vi "3.11-Select Critical Point.vi"(2 "Y (mm)":dbl[](array[numeric])=[-824.0, -821.8748054185536, -817.5016965016204, -818.8762184987505, -802.0414964088986, -800.9405372657634, -800.59012577146, -788.0816444032098, -786.2728465808068, -784.2245424325394, -781.9373558916932, -787.2650011250265, -784.474375788512, -778.521681763403, -776.2365810207972, -783.3658451204344, 730.5588889131224, 725.4102955430903, 724.8109075281693, 724.931328200215, 718.9384865393471, 714.6245895498994, 721.8640829579484, 720.0248002938554, 725.866494387571, 726.5437830014478, 731.9681149910491, 736.1878818898, 736.2022690917503, 745.9762624616667, 740.54860282115, 736.8877513302604, 737.0, -580.0, -600.0, -620.0, -640.0, -660.0, -680.0, -700.0, -720.0, -740.0, -760.0, -780.0, -800.0, -820.0, -840.0, -860.0, -880.0, -900.0, -920.0, -940.0, -960.0, -980.0, -1000.0, -1020.0, -1040.0, -1060.0, -1080.0, -1100.0, -1120.0, -1140.0, -1160.0, 580.0, 600.0, 620.0, 640.0, 660.0, 680.0, 700.0, 720.0, 740.0, 760.0, 780.0, 800.0, 820.0, 840.0, 860.0, 880.0, 900.0, 920.0, 940.0, 960.0, 980.0, 1000.0, 1020.0, 1040.0, 1060.0, 1080.0, 1100.0, 1120.0, 1140.0, 1160.0], 3 "X (mm)":dbl[](array[numeric])=[840.0, 854.3458780914469, 868.5477883026458, 882.9154841192139, 896.0842048902769, 910.0732171691171, 924.145412930461, 936.7642586636871, 950.5034421622921, 964.2089652419434, 977.8766530675427, 993.028814291989, 1006.7451760358431, 1019.7358924207481, 1033.5375164797342, 1049.9022455781442, 1049.4843904209192, 1034.373102871993, 1020.7156560129519, 1007.3635844318354, 992.8150927510532, 978.9089486341247, 967.2841142298599, 954.0407250143282, 942.0138830037281, 929.2083593725679, 916.9329489649929, 904.4080938905194, 891.4802776231645, 879.0949593134791, 865.8605270565532, 852.8624235442778, 840.0, 0.0, 0.0, 0.0, 0.0, 0.0, 0.0, 0.0, 0.0, 0.0, 0.0, 0.0, 0.0, 0.0, 0.0, 0.0, 0.0, 0.0, 0.0, 0.0, 0.0, 0.0, 0.0, 0.0, 0.0, 0.0, 0.0, 0.0, 0.0, 0.0, 0.0, 0.0, 0.0, 0.0, 0.0, 0.0, 0.0, 0.0, 0.0, 0.0, 0.0, 0.0, 0.0, 0.0, 0.0, 0.0, 0.0, 0.0, 0.0, 0.0, 0.0, 0.0, 0.0, 0.0, 0.0, 0.0, 0.0, 0.0, 0.0, 0.0, 0.0]) -> (0 "Left Data":T2, 1 "Right Data":T1)   [LabVIEW 2010]
panel:
  in  "Y (mm) 2":dbl[](array[numeric])
  in  "X (mm) 2":dbl[](array[numeric])
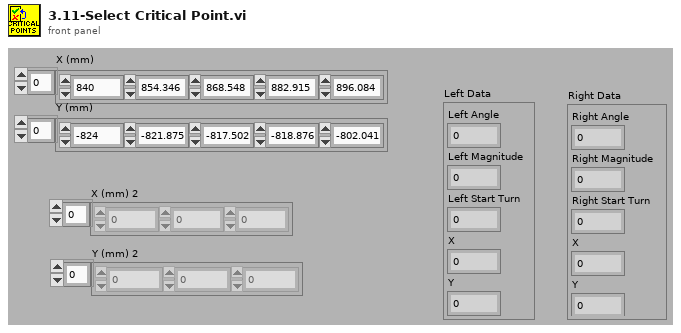
[diagram p1: front panel]
types:
  T1 = cluster{"Right Angle":dbl, "Right Magnitude":dbl, "Right Start Turn":dbl, "X":dbl, "Y":dbl}
  T2 = cluster{"Left Angle":dbl, "Left Magnitude":dbl, "Left Start Turn":dbl, "X":dbl, "Y":dbl}
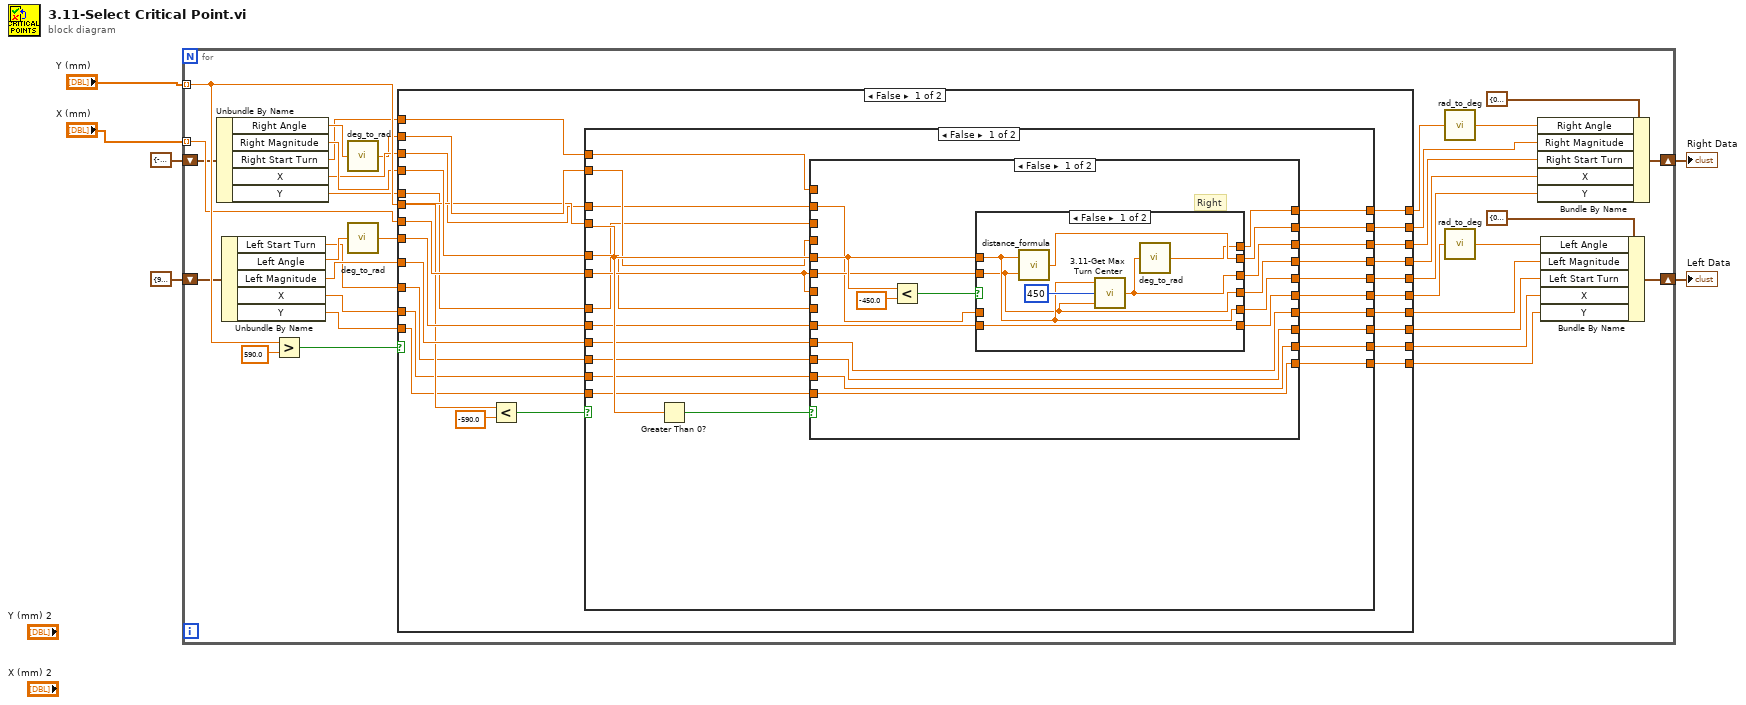
[diagram p0: block diagram]
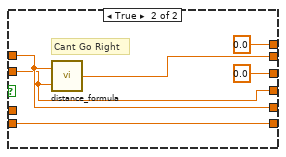
[diagram p2: hidden frame]
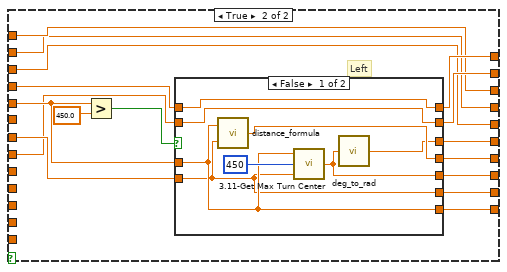
[diagram p3: hidden frame]
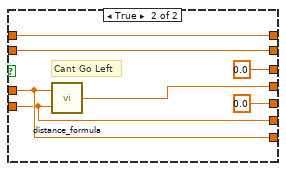
[diagram p4: hidden frame]
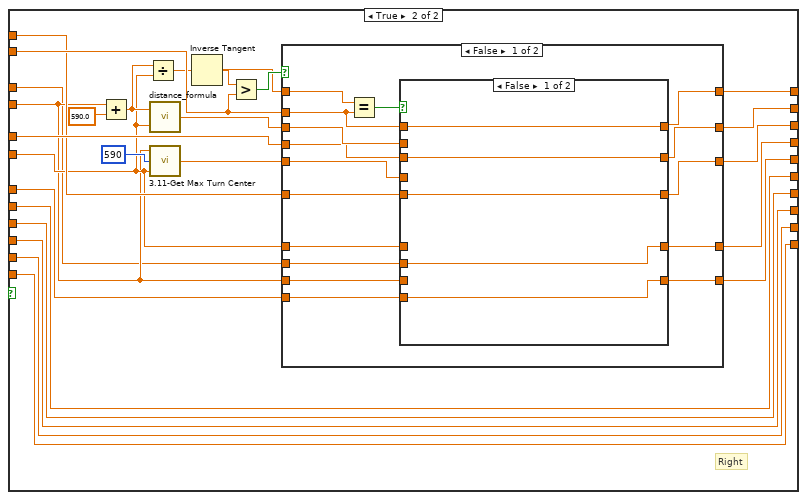
[diagram p5: hidden frame]
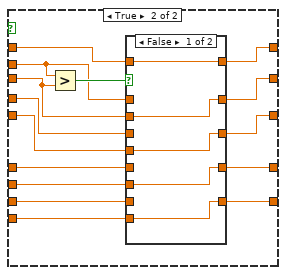
[diagram p6: hidden frame]
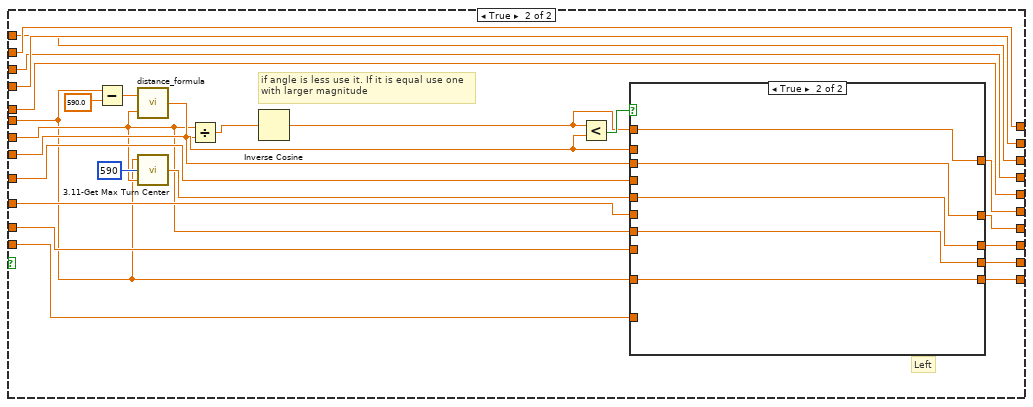
[diagram p9: hidden frame]
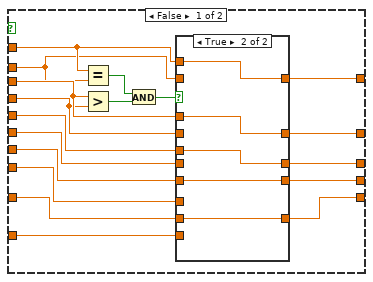
[diagram p10: hidden frame]
diagram:
  n1 = for {
    tunnel: "Y (mm)" -> [w38] mode=indexing
    tunnel: "X (mm)" -> [w37] mode=indexing
    shift-right: [w35] -> w3
    shift-left: T1 {"Right Angle"=-90.0, "Right Magnitude"=0.0, "Right Start Turn"=-90.0, "X"=-1.0, "Y"=-1701.0} ("input cluster") -> [w23]
    shift-right: [w21] -> w4
    shift-left: T2 {"Left Angle"=90.0, "Left Magnitude"=0.0, "Left Start Turn"=90.0, "X"=-1.0, "Y"=1701.0} ("input cluster") -> [w25]
    n2 = Unbundle By Name(w23) -> ("Right Angle"=w12:dbl, "Right Magnitude"=w22:dbl, "Right Start Turn"=w7:dbl, "X"=w15:dbl, "Y"=w13:dbl)
    n3 = Unbundle By Name(w25) -> ("Left Start Turn"=w8:dbl, "Left Angle"=w10:dbl, "Left Magnitude"=w24:dbl, "X"=w20:dbl, "Y"=w17:dbl)
    n4 = Greater?(x=w38, y=590.0) -> (0:w40:bool)
    n5 = call "deg_to_rad.vi"("Degrees"=w12) -> ("Radians"=w11:dbl)
    n6 = call "deg_to_rad.vi"("Degrees"=w10) -> ("Radians"=w9:dbl)
    n7 = case shown="False" w40 {
      tunnel: w38 -> [w53 w227]
      tunnel: w37 -> [w54 w229]
      tunnel: w9 -> [w62 w245]
      tunnel: [w61 w247] -> w29
      tunnel: [w59 w246] -> w26
      tunnel: w24 -> [w60 w244]
      tunnel: w11 -> [w58 w243]
      tunnel: [w57 w243] -> w32
      tunnel: [w55 w242] -> w33
      tunnel: w22 -> [w56 w242]
      tunnel: w8 -> [w49 w233]
      tunnel: [w50 w234] -> w27
      tunnel: [w52 w236] -> w34
      tunnel: w7 -> [w51 w236]
      tunnel: w20 -> [w42 w231]
      tunnel: [w41 w230] -> w19
      tunnel: [w44 w228] -> w18
      tunnel: w17 -> [w43 w226]
      tunnel: [w48 w225] -> w16
      tunnel: w15 -> [w47 w225]
      tunnel: [w46 w224] -> w14
      tunnel: w13 -> [w45 w224]
      frame False {
        n8 = Less?(x=w53, y=-590.0) -> (x < y?=w64:bool)
        n9 = case shown="False" w64 {
          tunnel: w62 -> [w83 w171]
          tunnel: [w85 w171] -> w61
          tunnel: w60 -> [w75 w170]
          tunnel: [w84 w170] -> w59
          tunnel: w58 -> [w79 w169]
          tunnel: [w82 w168] -> w57
          tunnel: w56 -> [w78 w166]
          tunnel: [w80 w167] -> w55
          tunnel: w54 -> [w81 w153]
          tunnel: w53 -> [w86 w152]
          tunnel: [w76 w159] -> w52
          tunnel: w51 -> [w73 w158]
          tunnel: [w77 w157] -> w50
          tunnel: w49 -> [w74 w157]
          tunnel: [w66 w155] -> w48
          tunnel: w47 -> [w72 w150]
          tunnel: [w67 w154] -> w46
          tunnel: w45 -> [w65 w151]
          tunnel: [w68 w148] -> w44
          tunnel: w43 -> [w69 w148]
          tunnel: [w71 w149] -> w41
          tunnel: w42 -> [w70 w149]
          frame False {
            n10 = Greater Than 0?(x=w86) -> (x > 0?=w87:bool)
            n11 = case shown="False" w87 {
              tunnel: w86 -> [w98 w129]
              tunnel: [w101 w130] -> w85
              tunnel: w81 -> [_ w128]
              tunnel: [w94 w127] -> w84
              tunnel: w83 -> [w100 _]
              tunnel: [w99 w126] -> w82
              tunnel: w81 -> [w97 _]
              tunnel: [w96 w124] -> w80
              tunnel: w79 -> [_ w125]
              tunnel: w78 -> [_ w123]
              tunnel: [w93 w122] -> w77
              tunnel: [w95 w121] -> w76
              tunnel: w75 -> [w94 _]
              tunnel: w74 -> [w93 _]
              tunnel: w73 -> [_ w121]
              tunnel: [w88 w117] -> w66
              tunnel: [w89 w118] -> w67
              tunnel: w72 -> [w92 w117]
              tunnel: [w91 w119] -> w71
              tunnel: w70 -> [w91 _]
              tunnel: w69 -> [w90 _]
              tunnel: [w90 w120] -> w68
              tunnel: w65 -> [_ w118]
              frame False {
                # "Right"
                n12 = Less?(x=w98, y=-450.0) -> (x < y?=w102:bool)
                n13 = case shown="False" w102 {
                  tunnel: [w109 w116] -> w101
                  tunnel: w100 -> [w109 w116]
                  tunnel: [w106 0.0 ("y")] -> w99
                  tunnel: w98 -> [w105 w112]
                  tunnel: w97 -> [w104 w111]
                  tunnel: [w108 w114] -> w96
                  tunnel: [w107 0.0 ("y")] -> w95
                  tunnel: w92 -> [_ _]
                  tunnel: [w105 w112] -> w89
                  tunnel: [w104 w111] -> w88
                  frame False {
                    n14 = call "distance_formula.vi"("X2 - X1"=w104, "Y2 - Y1"=w105) -> ("Distance"=w108:dbl)
                    n15 = call "3.11-Get Max Turn Center.vi"("X (mm)"=w104, "Distance Along Y where polar system is centered"=450, "Y (mm)"=w105) -> ("Start Turn Angle"=w107:dbl)
                    n16 = call "deg_to_rad.vi"("Degrees"=w107) -> ("Radians"=w106:dbl)
                  }
                  frame True {
                    # "Cant Go Right"
                    n17 = call "distance_formula.vi"("X2 - X1"=w111, "Y2 - Y1"=w112) -> ("Distance"=w114:dbl)
                  }
                }
              }
              frame True {
                # "Left"
                n18 = Greater?(x=w129, y=450.0) -> (0:w132:bool)
                n19 = case shown="False" w132 {
                  tunnel: [w135 0.0 ("y")] -> w130
                  tunnel: w129 -> [w134 w142]
                  tunnel: w128 -> [w133 w141]
                  tunnel: [w137 w146] -> w127
                  tunnel: [w139 w145] -> w126
                  tunnel: w125 -> [w139 w145]
                  tunnel: [w138 w144] -> w124
                  tunnel: w123 -> [w138 w144]
                  tunnel: [w136 0.0 ("y")] -> w122
                  tunnel: [w134 w142] -> w120
                  tunnel: [w133 w141] -> w119
                  frame False {
                    n20 = call "distance_formula.vi"("X2 - X1"=w133, "Y2 - Y1"=w134) -> ("Distance"=w137:dbl)
                    n21 = call "3.11-Get Max Turn Center.vi"("X (mm)"=w133, "Distance Along Y where polar system is centered"=450, "Y (mm)"=w134) -> ("Start Turn Angle"=w136:dbl)
                    n22 = call "deg_to_rad.vi"("Degrees"=w136) -> ("Radians"=w135:dbl)
                  }
                  frame True {
                    # "Cant Go Left"
                    n23 = call "distance_formula.vi"("X2 - X1"=w141, "Y2 - Y1"=w142) -> ("Distance"=w146:dbl)
                  }
                }
              }
            }
          }
          frame True {
            # "Right"
            n24 = Add(x=w152, y=590.0) -> (x+y=w162:dbl)
            n25 = Divide(x=w162, y=w153) -> (x/y=w163:dbl)
            n26 = call "distance_formula.vi"("X2 - X1"=w153, "Y2 - Y1"=w162) -> ("Distance"=w164:dbl)
            n27 = call "3.11-Get Max Turn Center.vi"("X (mm)"=w153, "Distance Along Y where polar system is centered"=590, "Y (mm)"=w152) -> ("Start Turn Angle"=w160:dbl)
            n28 = Inverse Tangent(1:w163) -> (0:w161:dbl)
            n29 = Greater?(x=w161, y=w169) -> (0:w172:bool)
            n30 = case shown="False" w172 {
              tunnel: w169 -> [w186 _]
              tunnel: w164 -> [w187 w223]
              tunnel: [w185 w222] -> w168
              tunnel: [w184 w223] -> w167
              tunnel: w166 -> [w183 _]
              tunnel: w161 -> [w182 w222]
              tunnel: [w181 w221] -> w159
              tunnel: w160 -> [w179 w221]
              tunnel: w158 -> [w180 _]
              tunnel: [w178 w220] -> w155
              tunnel: w153 -> [w177 w220]
              tunnel: [w176 w219] -> w154
              tunnel: w152 -> [w175 w219]
              tunnel: w151 -> [w174 _]
              tunnel: w150 -> [w173 _]
              frame False {
                n31 = Equal?(x=w182, y=w186) -> (x = y?=w188:bool)
                n32 = case shown="False" w188 {
                  tunnel: w187 -> [_ w203]
                  tunnel: w183 -> [w193 w207]
                  tunnel: w186 -> [w192 w206]
                  tunnel: [w192 w205] -> w185
                  tunnel: [w193 w204] -> w184
                  tunnel: [w191 w201] -> w181
                  tunnel: w180 -> [w191 w200]
                  tunnel: w179 -> [_ w202]
                  tunnel: [w189 w199] -> w178
                  tunnel: w177 -> [_ w198]
                  tunnel: [w190 w197] -> w176
                  tunnel: w175 -> [_ w196]
                  tunnel: w174 -> [w190 w195]
                  tunnel: w173 -> [w189 w194]
                  frame False {
                  }
                  frame True {
                    n33 = Greater?(x=w203, y=w207) -> (0:w208:bool)
                    n34 = case shown="False" w208 {
                      tunnel: w207 -> [w212 _]
                      tunnel: w206 -> [w213 w217]
                      tunnel: [w213 w217] -> w205
                      tunnel: [w212 w218] -> w204
                      tunnel: w203 -> [_ w218]
                      tunnel: [w211 w216] -> w201
                      tunnel: w202 -> [_ w216]
                      tunnel: w200 -> [w211 _]
                      tunnel: [w209 w215] -> w199
                      tunnel: w198 -> [_ w215]
                      tunnel: [w210 w214] -> w197
                      tunnel: w196 -> [_ w214]
                      tunnel: w195 -> [w210 _]
                      tunnel: w194 -> [w209 _]
                      frame False {
                      }
                      frame True {
                      }
                    }
                  }
                }
              }
              frame True {
              }
            }
          }
        }
      }
      frame True {
        # "if angle is less use it. If it is equal use one\nwith larger magnitude"
        # "Left"
        n35 = Subtract(x=w227, y=590.0) -> (x-y=w240:dbl)
        n36 = call "distance_formula.vi"("X2 - X1"=w229, "Y2 - Y1"=w240) -> ("Distance"=w238:dbl)
        n37 = call "3.11-Get Max Turn Center.vi"("X (mm)"=w229, "Distance Along Y where polar system is centered"=590, "Y (mm)"=w227) -> ("Start Turn Angle"=w235:dbl)
        n38 = Divide(x=w229, y=w238) -> (x/y=w239:dbl)
        n39 = Inverse Cosine(1:w239) -> (0:w237:dbl)
        n40 = Less?(x=w237, y=w245) -> (x < y?=w248:bool)
        n41 = case shown="True" w248 {
          tunnel: w237 -> [w261 w281]
          tunnel: [w260 w281] -> w247
          tunnel: w238 -> [w263 w280]
          tunnel: [w262 w280] -> w246
          tunnel: w245 -> [w259 _]
          tunnel: w244 -> [w258 _]
          tunnel: w235 -> [w255 w279]
          tunnel: [w256 w279] -> w234
          tunnel: w233 -> [w257 _]
          tunnel: w231 -> [w250 _]
          tunnel: [w252 w278] -> w230
          tunnel: w229 -> [w251 w278]
          tunnel: [w254 w277] -> w228
          tunnel: w227 -> [w253 w277]
          tunnel: w226 -> [w249 _]
          frame False {
            n42 = Equal?(x=w261, y=w259) -> (x = y?=w265:bool)
            n43 = Greater?(x=w263, y=w258) -> (0:w266:bool)
            n44 = And(x=w265, y=w266) -> (x .and. y?=w264:bool)
            n45 = case shown="True" w264 {
              tunnel: w263 -> [_ w276]
              tunnel: [w270 w276] -> w262
              tunnel: w261 -> [_ w275]
              tunnel: [w271 w275] -> w260
              tunnel: w259 -> [w271 _]
              tunnel: w258 -> [w270 _]
              tunnel: w257 -> [w269 _]
              tunnel: [w269 w274] -> w256
              tunnel: w255 -> [_ w274]
              tunnel: [w267 w273] -> w254
              tunnel: w253 -> [_ w273]
              tunnel: [w268 w272] -> w252
              tunnel: w251 -> [_ w272]
              tunnel: w250 -> [w268 _]
              tunnel: w249 -> [w267 _]
              frame False {
              }
              frame True {
              }
            }
          }
          frame True {
          }
        }
      }
    }
    n46 = call "rad_to_deg.vi"("Radians"=w32) -> ("Degrees"=w31:dbl)
    n47 = call "rad_to_deg.vi"("Radians"=w29) -> ("Degrees"=w28:dbl)
    n48 = Bundle By Name(cluster=T1 {"Right Angle"=0.0, "Right Magnitude"=0.0, "Right Start Turn"=0.0, "X"=450.0, "Y"=450.0} ("input cluster"), "Right Angle"=w31, "Right Magnitude"=w33, "Right Start Turn"=w34, "X"=w16, "Y"=w14) -> (w35:T1)
    n49 = Bundle By Name(cluster=T2 {"Left Angle"=0.0, "Left Magnitude"=0.0, "Left Start Turn"=0.0, "X"=0.0, "Y"=0.0} ("input cluster"), "Left Angle"=w28, "Left Magnitude"=w26, "Left Start Turn"=w27, "X"=w19, "Y"=w18) -> (w21:T2)
  }
  "Left Data" <- w4
  "Right Data" <- w3
